vi "Read Families.vi"(8 "error in (no error)":errorcluster, 11 "Parameters in":refnum<class "Parameters.lvclass">) -> (0 "error out":errorcluster, 2 "Families":T1[](array[typedef]), 3 "Parameters out":refnum<class "Parameters.lvclass">)   [LabVIEW 2020, in "Parameters.lvclass"]
uses:
  Parameters.lvclass
  Typedefs/Tosca-Parameter Family.ctl
  Typedefs/Tosca-Parameter Table Element.ctl
  Typedefs/Tosca-Parameter Dimension.ctl
  Parameters.lvclass/Parameters.ctl
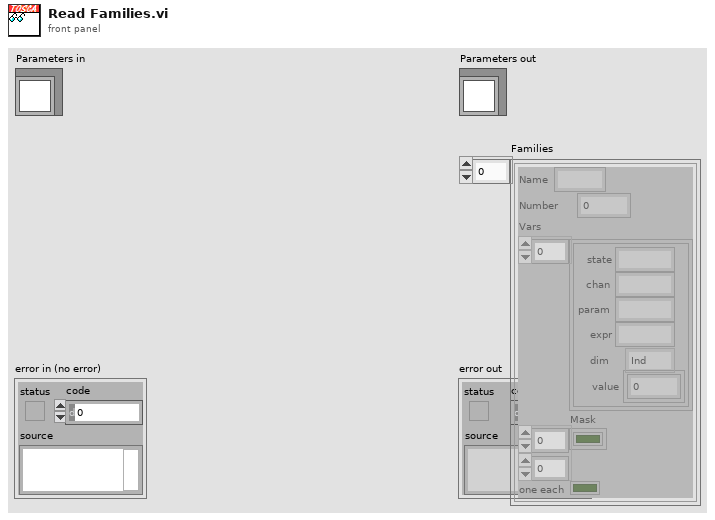
[diagram p1: front panel]
types:
  T1 = typedef "Tosca-Parameter Family.ctl" = cluster{"Name":string, "Number":i32, "Vars":T2[], "Mask":bool[][], "one each":bool}
  T2 = typedef "Tosca-Parameter Table Element.ctl" = cluster{"state":string, "chan":string, "param":string, "expr":string, "dim":T3, "value":dbl[]}
  T3 = typedef "Tosca-Parameter Dimension.ctl" = enum16{"Ind", "X", "Y"}
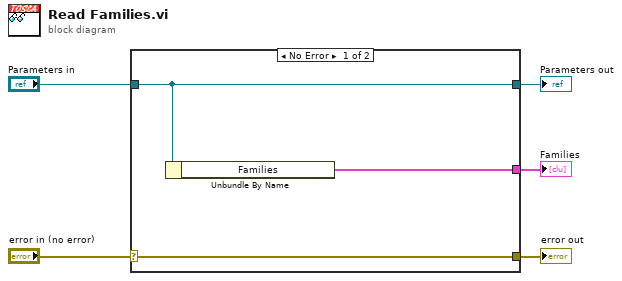
[diagram p0: block diagram]
diagram:
  n1 = case shown="No Error" "error in (no error)" {
    selector: "error in (no error)" -> [w8 w9]
    tunnel: [w8 w9] -> w4
    tunnel: [w7 w10] -> w2
    tunnel: "Parameters in" -> [w7 w10]
    tunnel: [w6 _] -> w1
    frame No Error {
      n2 = Unbundle By Name(w7) -> ("Families"=w6:T1[])
    }
    frame Error {
    }
  }
  "error out" <- w4
  "Parameters out" <- w2
  "Families" <- w1
